vi "SqGn SD Load Steps from Sequence.vi"(8 "error in (no error)":errorcluster, 10 "Sequence":refnum<k7>, 11 "SeqGen Step Dictionary in":refnum<class "SeqGen Step Dictionary.lvclass">) -> (0 "error out":errorcluster, 2 "Sequence Reference Out":refnum<k7>, 3 "SeqGen Step Dictionary out":refnum<class "SeqGen Step Dictionary.lvclass">)   [LabVIEW 2018, in "SeqGen Step Database.lvlib" / "SeqGen Step Dictionary.lvclass"]
uses:
  SeqGen Step Dictionary.lvclass
  Plugins/TestStand API Tools (TSAT).lvlibp/Sequence Actions/TSAT Sequence Actions.lvlib
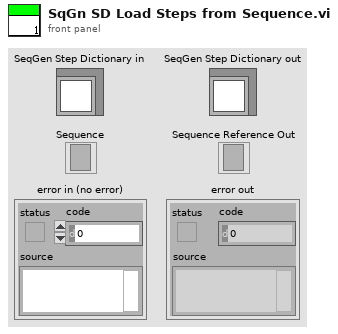
[diagram p1: front panel]
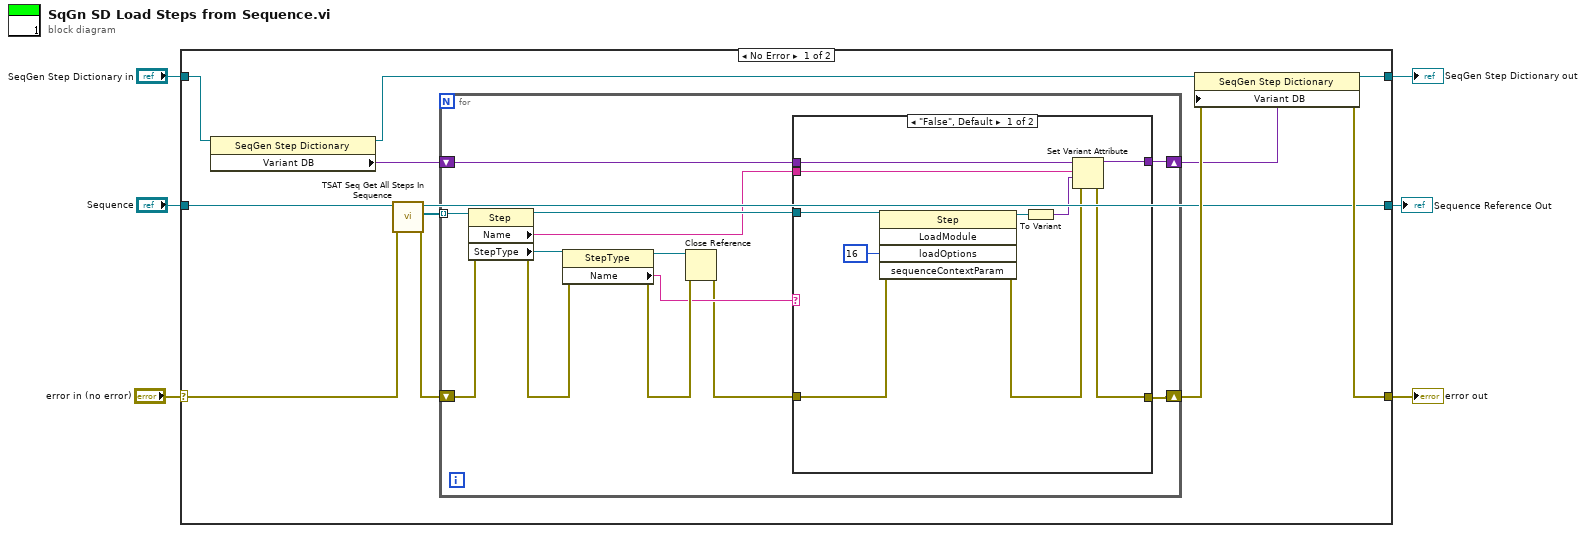
[diagram p0: block diagram]
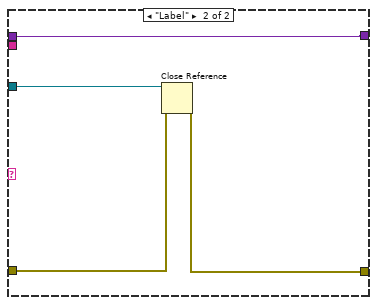
[diagram p2: hidden frame]
diagram:
  n1 = case shown="No Error" "error in (no error)" {
    selector: "error in (no error)" -> [w16 w48]
    tunnel: [w11 w48] -> w5
    tunnel: [w9 w47] -> w3
    tunnel: "SeqGen Step Dictionary in" -> [w18 w47]
    tunnel: "Sequence" -> [w17 w46]
    tunnel: [w7 w46] -> w1
    frame No Error {
      n2 = property class="SeqGen Step Dictionary"(reference=w18) -> (reference out=w10:refnum<class "SeqGen Step Dictionary.lvclass">, "Variant DB"=w12:variant)  [unwired: 1 in, 1 out]
      n3 = call "TSAT Seq Get All Steps In Sequence.vi"("Error In"=w16, "Sequence Reference In"=w17) -> ("Error Out"=w15:errorcluster, "All Steps"=w14:refnum<k7>[], "Sequence Reference Out"=w7:refnum<k7>)  [unwired: 7 in]
      n4 = for {
        shift-right: [w23] -> w13
        shift-left: w15 -> [w29]
        tunnel: w14 -> [w31] mode=indexing
        shift-right: [w19] -> w8
        shift-left: w12 -> [w21]
        n5 = property class="Step"(reference=w31, error in=w29) -> (reference out=w22:refnum<k7>, error out=w28:errorcluster, "Name"=w20:string, "StepType"=w30:refnum<k7>)
        n6 = property class="StepType"(reference=w30, error in=w28) -> (reference out=w27:refnum<k7>, error out=w26:errorcluster, "Name"=w25:string)
        n7 = Close Reference(reference=w27, error in (no error)=w26) -> (error out=w24:errorcluster)
        n8 = case shown="\"False\", Default" w25 {
          tunnel: w24 -> [w40 w45]
          tunnel: [w35 w44] -> w23
          tunnel: w22 -> [w41 w43]
          tunnel: w21 -> [w38 w42]
          tunnel: w20 -> [w34 _]
          tunnel: [w33 w42] -> w19
          frame "False", Default {
            n9 = invoke class="Step" method="LoadModule"(reference=w41, error in=w40, "loadOptions"=16) -> (reference out=w39:refnum<k7>, error out=w36:errorcluster)  [unwired: 2 in, 3 out]
            n10 = To Variant(anything=w39) -> (Variant=w37:variant)
            n11 = Set Variant Attribute(Variant=w38, name=w34, value=w37, error in=w36) -> (Variant out=w33:variant, error out=w35:errorcluster)  [unwired: 1 out]
          }
          frame "Label" {
            n12 = Close Reference(reference=w43, error in (no error)=w45) -> (error out=w44:errorcluster)
          }
        }
      }
      n13 = property class="SeqGen Step Dictionary"(reference=w10, error in=w13, "Variant DB"=w8) -> (reference out=w9:refnum<class "SeqGen Step Dictionary.lvclass">, error out=w11:errorcluster)
    }
    frame Error {
    }
  }
  "error out" <- w5
  "SeqGen Step Dictionary out" <- w3
  "Sequence Reference Out" <- w1
